vi "Unequal_Safe_1dDBL.vi"(5 "x":dbl[](array[numeric]), 9 "y":dbl[](array[numeric])) -> (8 "Diff?":bool, 14 "Diff? array":bool[](array[boolean]))   [LabVIEW 2013]
doc: "Assesses x not equal to y?, up to length of x. The output 'which diff?' always matches the length of x. Additionally, 'diff?' is provided for convenience as the array-OR for a simple boolean indicating at lease one difference."
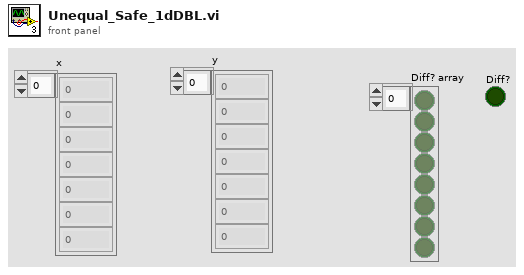
[diagram p1: front panel]
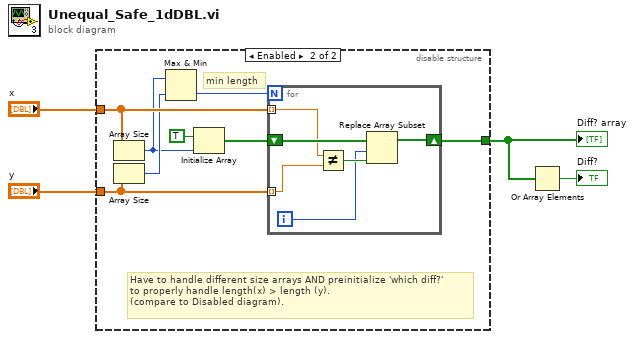
[diagram p0: block diagram]
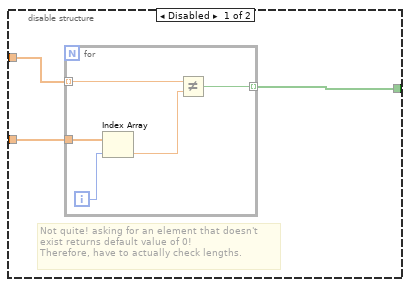
[diagram p2: hidden frame]
diagram:
  n1 = disable-structure shown="Enabled" {
    disable-tunnel: "x" -> [w7 w17]
    disable-tunnel: "y" -> [w6 w18]
    disable-tunnel: [w5 w13] -> w2
    frame Disabled {
      # "Not quite! asking for an element that doesn't \nexist returns default value of 0!\nTherefore, have to actually check lengths."
      n2 = for {
        tunnel: w7 -> [w10] mode=indexing
        tunnel: w6 -> [w12]
        tunnel: [w8] -> w5 mode=indexing
        i -> [w11]
        n3 = Index Array(array=w12, index=w11) -> (element=w9:dbl)
        n4 = Not Equal?(x=w10, y=w9) -> (x != y?=w8:bool)
      }
    }
    frame Enabled {
      # "Have to handle different size arrays AND preinitialize 'which diff?'\nto properly handle length(x) > length (y).\n(compare to Disabled diagram)."
      # "min length"
      n5 = Array Size(array=w17) -> (size(s)=w15:i32)
      n6 = Array Size(array=w18) -> (size(s)=w16:i32)
      n7 = Max & Min(x=w15, y=w16) -> (min(x,y)=w14:i32)  [unwired: 1 out]
      n8 = Initialize Array(TRUE, w15) -> (w19:bool[])
      n9 = for {
        N: w14 -> [_]
        shift-right: [w25] -> w13
        shift-left: w19 -> [w26]
        tunnel: w18 -> [w22] mode=indexing
        tunnel: w17 -> [w23] mode=indexing
        i -> [w21]
        n10 = Not Equal?(x=w23, y=w22) -> (x != y?=w24:bool)
        n11 = Replace Array Subset(array=w26, new element=w24, index=w21) -> (w25:bool[])
      }
    }
  }
  "Diff? array" <- w2
  n12 = Or Array Elements(Boolean array=w2) -> (logical OR=→"Diff?":bool)
